vi "01 - Varied Math Libraries.vi"() -> ()   [LabVIEW 2021]
uses:
  <vilib>/Analysis/NI_AALPro.lvlib
  <vilib>/gmath/NI_Gmath.lvlib
  <vilib>/Analysis/NI_AALBase.lvlib
  <vilib>/gmath/statdist.llb/Rayleigh Random.vi
  <vilib>/gmath/interp.llb/Interpolate 2D (2d X,Y).vi
  <vilib>/Analysis/coordinate.llb/3D Cartesian Coordinate Rotation (Euler) (Array).vi
  <vilib>/Analysis/7linalg.llb/Solve Linear Equations (single right hand).vi
  <vilib>/Analysis/polynomials.llb/Polynomial Roots (DBL).vi
  <vilib>/Analysis/baseanly.llb/Matrix Type of Inverse Matrix.ctl
  <vilib>/Analysis/Matrix/Datatypes/RealMatrix.ctl
  <vilib>/Analysis/Matrix/NI_Matrix.lvlib
panel:
  out "transposed matrix":T1
  out "Solution Vector":dbl[](array[numeric]) format="%.2f"
  out "error":i32
  in  "Input Matrix":T1
  in  "Known Vector":dbl[](array[numeric]) format="%.2f"
  in  "matrix type":T2
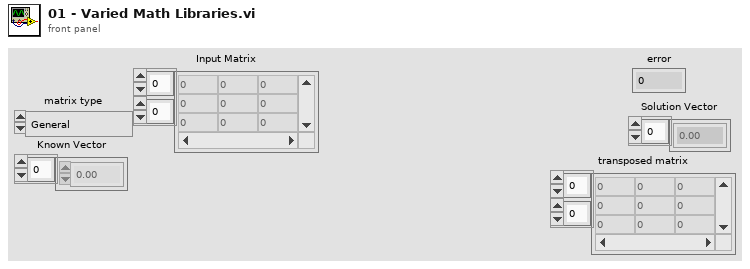
[diagram p1: front panel]
types:
  T1 = typedef "NI_Matrix.lvlib/RealMatrix.ctl" = dbl[][]
  T2 = typedef "NI_AALBase.lvlib/Matrix Type of Inverse Matrix.ctl" = enum32{"General", "Positive Definite", "Lower Triangular", "Upper Triangular"}
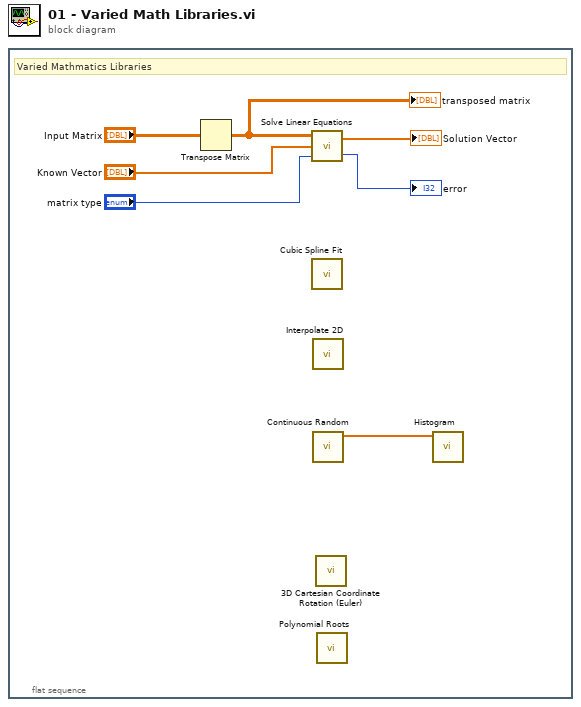
[diagram p0: block diagram]
diagram:
  n1 = flat-sequence {
    frame #0 {
      # "Varied Mathmatics Libraries"
      n2 = Transpose Matrix(1:"Input Matrix") -> (0:w2:T1)
      "transposed matrix" <- w2
      n3 = call-poly <vilib>:"Solve Linear Equations.vi"("matrix type"="matrix type", "Known Vector"="Known Vector", "Input Matrix"=w2) -> ("error"=→"error":i32, "Solution Vector"=→"Solution Vector":dbl[])
      n4 = call <vilib>:"Cubic Spline Fit.vi"() -> ()  [unwired: 14 in, 2 out]
      n5 = call-poly <vilib>:"Interpolate 2D.vi"() -> ()  [unwired: 8 in, 4 out]
      n6 = call-poly <vilib>:"Continuous Random.vi"() -> ("Rayleigh random data"=w1:dbl[])  [unwired: 10 in, 1 out]
      n7 = call-poly <vilib>:"3D Cartesian Coordinate Rotation (Euler).vi"() -> ()  [unwired: 8 in, 4 out]
      n8 = call-poly <vilib>:"Polynomial Roots.vi"() -> ()  [unwired: 10 in, 2 out]
      n9 = call <vilib>:"Histogram.vi"("X"=w1) -> ()  [unwired: 7 in, 4 out]
    }
  }
